vi "SPI_Get_Number_Of_Devices.vi"() -> (0 "NumDevices":u32, 1 "FTC_Status":u32)   [LabVIEW 2010]
uses:
  WINNT/system32/FTCSPI.dll
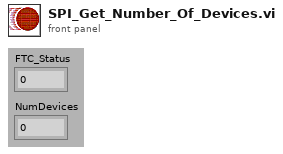
[diagram p1: front panel]
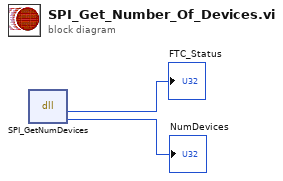
[diagram p0: block diagram]
diagram:
  n1 = dll-call lib="C:/Users/WINNT/system32/FTCSPI.dll" fn="SPI_GetNumDevices"() -> ("FTC_Status"=→"FTC_Status":u32, "NumDevices"=→"NumDevices":u32)  [unwired: 4 in, 2 out]
